vi "load_waveform_xml.vi"(8 "error (in)":errorcluster, 11 "Node (in)":refnum<k20>) -> (0 "error":errorcluster, 1 "Waveform prototype":T1, 3 "Node":refnum<k20>)   [LabVIEW 2013]
uses:
  waveform.ctl
  Globals.vi
  <vilib>/xml/Close Reference(Node).vi
  HSDIO.lvclass
  <resource>/objmgr/DOMUserDefRef.rc
  <vilib>/xml/NI_XML.lvlib
panel:
  out "array":u8[][](array[numeric])
  out "node text":string
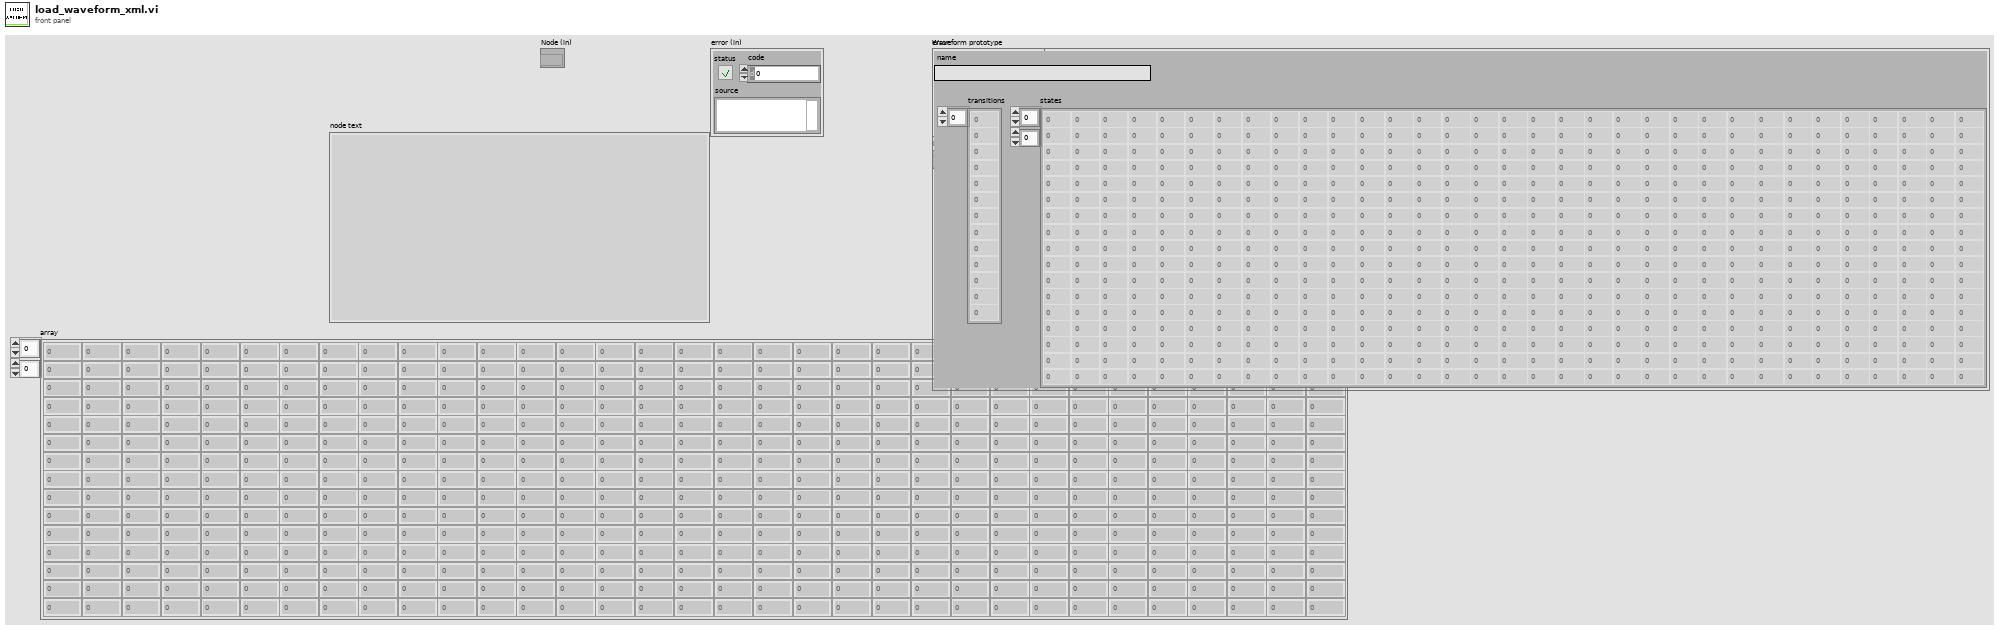
[diagram p1: front panel]
types:
  T1 = typedef "HSDIO.lvclass/waveform.ctl" = cluster{"name":string, "transitions":u32[], "states":u8[][]}
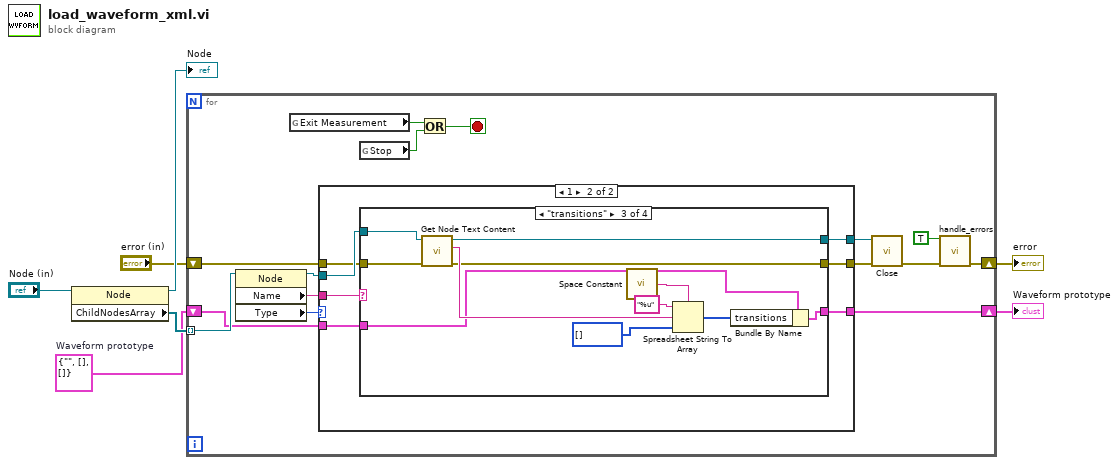
[diagram p0: block diagram]
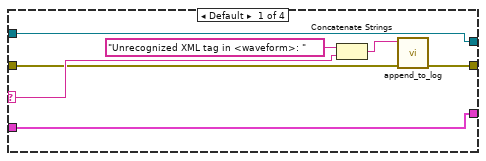
[diagram p3: hidden frame]
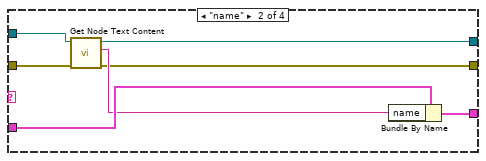
[diagram p4: hidden frame]
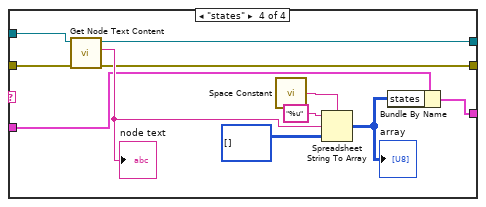
[diagram p5: hidden frame]
diagram:
  w3 = T1 {"name"="", "transitions"=[], "states"=[]}  # Waveform prototype
  n1 = property class="Node"(reference="Node (in)") -> (reference out=→"Node":refnum<k20>, "ChildNodesArray"=w4:refnum<k20>[])  [unwired: 1 in, 1 out]
  n2 = for {
    tunnel: w4 -> [w22] mode=indexing
    shift-right: [w19] -> w5
    shift-left: w3 -> [w20]
    shift-right: [w10] -> w7
    shift-left: "error (in)" -> [w16]
    stop <- w9 stop-if-true
    n3 = property class="Node"(reference=w22) -> (reference out=w18:refnum<k20>, "Name"=w21:string, "Type"=w8:i32)  [unwired: 1 in, 1 out]
    n4 = global read "Globals.vi" "Exit Measurement"() -> (w13:bool)
    n5 = case shown="1" w8 {
      tunnel: w21 -> [_ w32]
      tunnel: w20 -> [w23 w31]
      tunnel: [w23 w30] -> w19
      tunnel: w18 -> [w24 w29]
      tunnel: [w24 w28] -> w17
      tunnel: w16 -> [w25 w27]
      tunnel: [w25 w26] -> w15
      frame 0, Default {
      }
      frame 1 {
        n6 = case shown="\"transitions\"" w32 {
          selector: w32 -> [w35 _ _ _]
          tunnel: w31 -> [w38 w46 w53 w64]
          tunnel: [w38 w45 w52 w63] -> w30
          tunnel: w29 -> [w39 w44 w50 w61]
          tunnel: [w39 w43 w51 w62] -> w28
          tunnel: w27 -> [w34 w42 w49 w60]
          tunnel: [w33 w40 w48 w59] -> w26
          frame Default {
            n7 = Concatenate Strings("Unrecognized XML tag in <waveform>: " ("string"), w35) -> (w36:string)
            n8 = call "append_to_log.vi"("error in"=w34, "string"=w36) -> ("error out"=w33:errorcluster)  [unwired: 9 in]
          }
          frame "name" {
            n9 = call <vilib>:"Get Node Text Content.vi"("error in (no error)"=w42, "node in"=w44) -> ("error out"=w40:errorcluster, "node text"=w41:string, "node out"=w43:refnum<k20>)  [unwired: 7 in]
            n10 = Bundle By Name(cluster=w46, "name"=w41) -> (w45:T1)
          }
          frame "transitions" {
            n11 = call <vilib>:"Get Node Text Content.vi"("error in (no error)"=w49, "node in"=w50) -> ("error out"=w48:errorcluster, "node text"=w55:string, "node out"=w51:refnum<k20>)  [unwired: 7 in]
            n12 = call <vilib>:"Space Constant.vi"() -> ("String"=w47:string)
            n13 = Spreadsheet String To Array(delimiter (Tab)=w47, format string="%u", spreadsheet string=w55, array type (2D Dbl)=u32[] []) -> (array=w54:u32[])
            n14 = Bundle By Name(cluster=w53, "transitions"=w54) -> (w52:T1)
          }
          frame "states" {
            n15 = call <vilib>:"Get Node Text Content.vi"("error in (no error)"=w60, "node in"=w61) -> ("error out"=w59:errorcluster, "node text"=w66:string, "node out"=w62:refnum<k20>)  [unwired: 7 in]
            "node text" <- w66
            n16 = call <vilib>:"Space Constant.vi"() -> ("String"=w58:string)
            n17 = Spreadsheet String To Array(delimiter (Tab)=w58, format string="%u", spreadsheet string=w66, array type (2D Dbl)=u8[][] []) -> (array=w65:u8[][])
            "array" <- w65
            n18 = Bundle By Name(cluster=w64, "states"=w65) -> (w63:T1)
          }
        }
      }
    }
    n19 = global read "Globals.vi" "Stop"() -> (w14:bool)
    n20 = Or(x=w13, y=w14) -> (x .or. y?=w9:bool)
    n21 = call-poly <vilib>:"Close.vi"("error in (no error)"=w15, "node"=w17) -> ("error out"=w11:errorcluster)  [unwired: 7 in]
    n22 = call "handle_errors.vi"("Exit Operation"=TRUE ("Exit Measurement"), "error in (no error)"=w11) -> ("error out"=w10:errorcluster)  [unwired: 13 in]
  }
  "error" <- w7
  "Waveform prototype" <- w5
